vi "camera decode TCP.vi"(9 "Numeric":u32) -> (1 "camera commands":string[](array[string]))   [LabVIEW 2021]
panel:
  out "command 1":string
  out "Array 1":u8[](array[numeric])
  out "command 2":string
  out "Array 2":u8[](array[numeric])
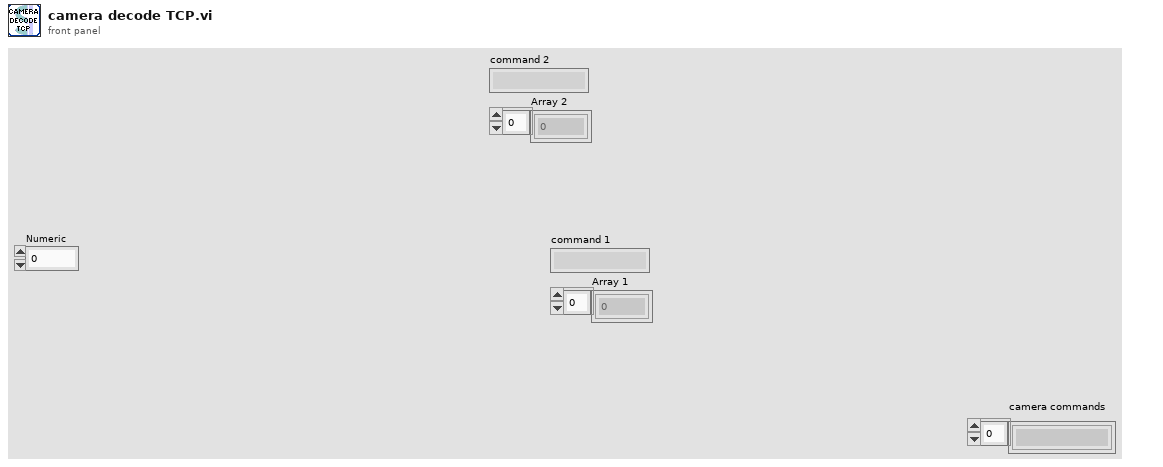
[diagram p1: front panel]
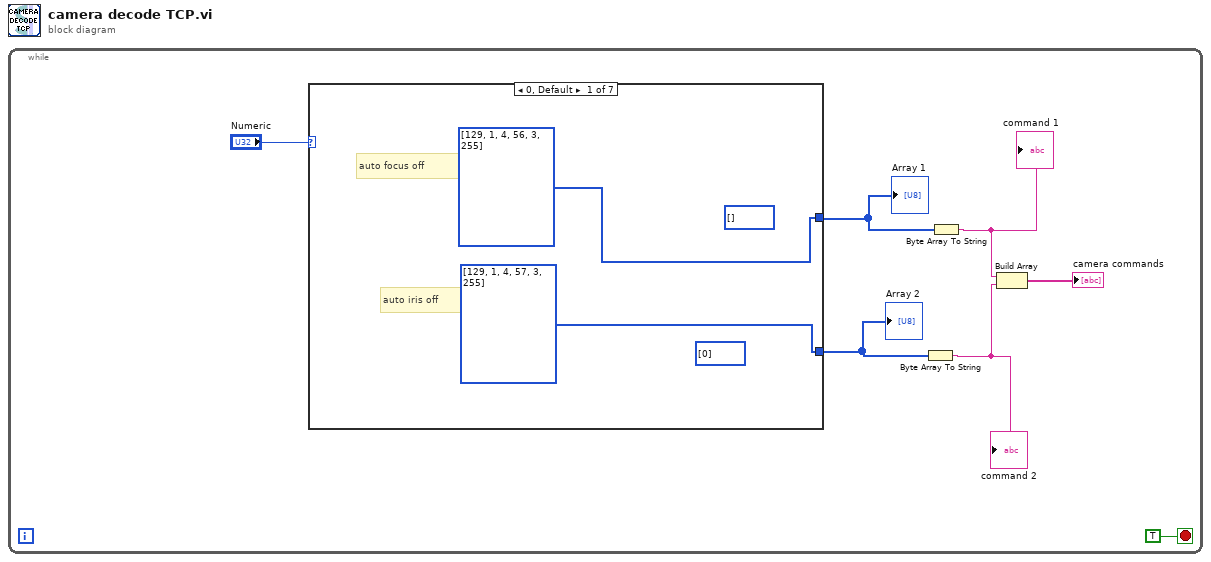
[diagram p0: block diagram]
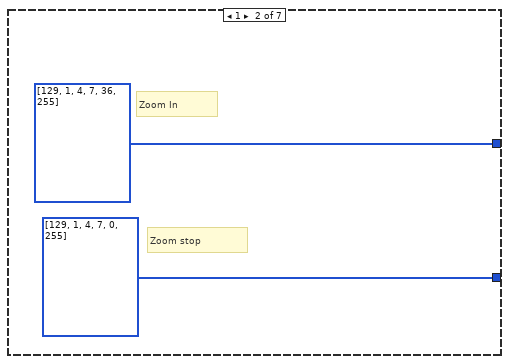
[diagram p2: hidden frame]
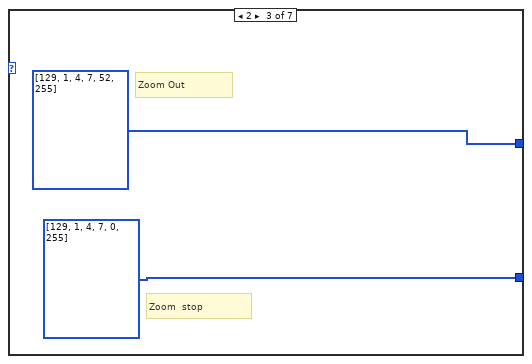
[diagram p3: hidden frame]
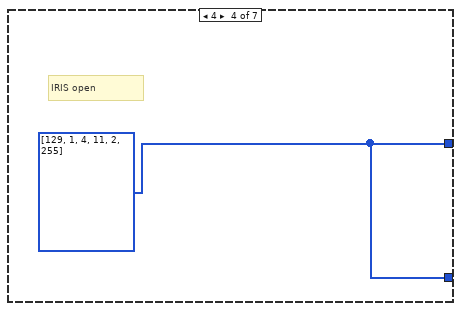
[diagram p4: hidden frame]
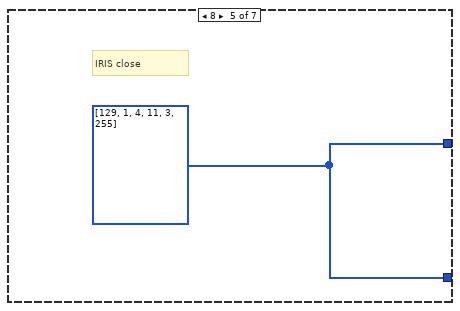
[diagram p5: hidden frame]
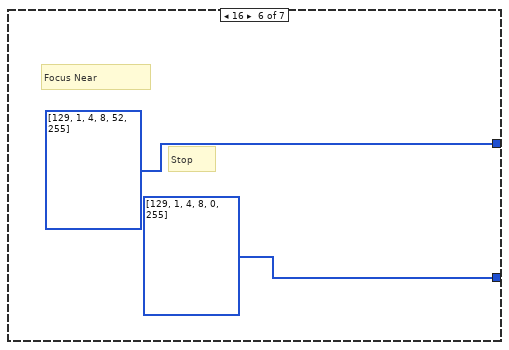
[diagram p6: hidden frame]
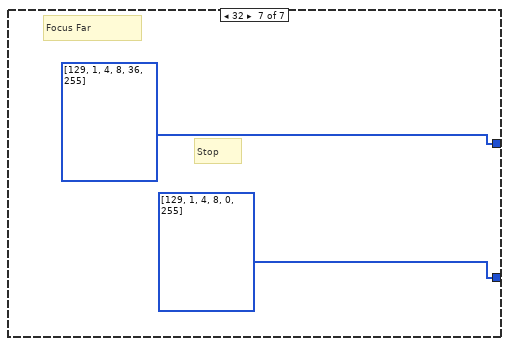
[diagram p7: hidden frame]
diagram:
  n1 = while {
    stop <- TRUE stop-if-true
    n2 = case shown="0, Default" "Numeric" {
      tunnel: [u8[] [129, 1, 4, 56, 3, 255] u8[] [129, 1, 4, 7, 36, 255] u8[] [129, 1, 4, 7, 52, 255] w14 w15 u8[] [129, 1, 4, 8, 52, 255] u8[] [129, 1, 4, 8, 36, 255]] -> w5
      tunnel: [u8[] [129, 1, 4, 57, 3, 255] u8[] [129, 1, 4, 7, 0, 255] u8[] [129, 1, 4, 7, 0, 255] w14 w15 u8[] [129, 1, 4, 8, 0, 255] u8[] [129, 1, 4, 8, 0, 255]] -> w4
      frame 0, Default {
        (unwired) u8[] [0]
        (unwired) u8[] []
        # "auto iris off"
        # "auto focus off"
      }
      frame 1 {
        # "Zoom stop"
        # "Zoom In"
      }
      frame 2 {
        # "Zoom  stop"
        # "Zoom Out"
      }
      frame 4 {
        w14 = u8[] [129, 1, 4, 11, 2, 255]
        # "IRIS open"
      }
      frame 8 {
        w15 = u8[] [129, 1, 4, 11, 3, 255]
        # "IRIS close"
      }
      frame 16 {
        # "Stop"
        # "Focus Near"
      }
      frame 32 {
        # "Stop"
        # "Focus Far"
      }
    }
    "Array 1" <- w5
    "Array 2" <- w4
    n3 = Byte Array To String(unsigned byte array=w4) -> (string=w2:string)
    "command 2" <- w2
    n4 = Byte Array To String(unsigned byte array=w5) -> (string=w3:string)
    "command 1" <- w3
    n5 = Build Array(w3, w2) -> (→"camera commands":string[])
  }
